vi "NB_GetProperty.vi"(0 "object in":refnum<class "NativeBaseTemplate.lvclass">, 5 "Error In":errorcluster) -> (14 "object out":refnum<class "NativeBaseTemplate.lvclass">, 15 "property":bool, 19 "Error Out":errorcluster)   [LabVIEW 2020, in "NativeBaseTemplate.lvclass"]
uses:
  <resource>/Framework/Providers/Open_GDS/ClassProviders/Provider_LvNativeClass/Templates/NativeBaseTemplate/NativeBaseTemplate.lvclass
  <resource>/Framework/Providers/Open_GDS/ClassProviders/Provider_LvNativeClass/Templates/NativeBaseTemplate/NativeBaseTemplate.lvclass/NativeBaseTemplate.ctl
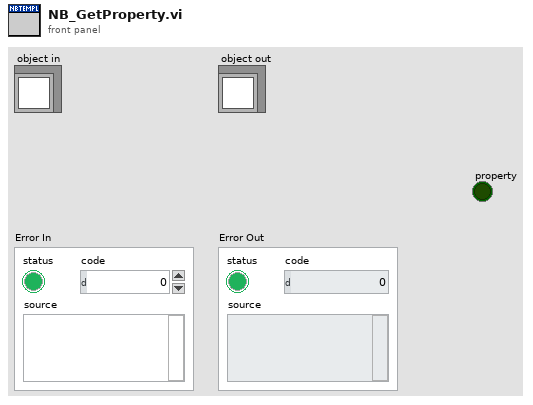
[diagram p1: front panel]
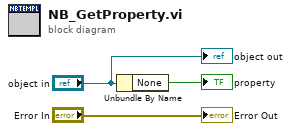
[diagram p0: block diagram]
diagram:
  n1 = Unbundle By Name("object in") -> ("None"=→"property":bool)
  "Error Out" <- "Error In"
  "object out" <- "object in"
